vi "PLC_OP10_Read.vi"(8 "error in (no error)":errorcluster, 11 "S7 Connection in":T1) -> (0 "error out":errorcluster, 3 "S7 Connection out":T1)   [LabVIEW 2017]
uses:
  <vilib>/DATA AHEAD/SP7/typedefs/S7 Connection.ctl
  <vilib>/DATA AHEAD/SP7/typedefs/PLC Type.ctl
  <vilib>/DATA AHEAD/SP7/functions/read/read real array.vi
  <vilib>/DATA AHEAD/SP7/functions/read/read String.vi
  <vilib>/DATA AHEAD/SP7/functions/read/read Dint array.vi
  <vilib>/DATA AHEAD/SP7/SP7.lvlib
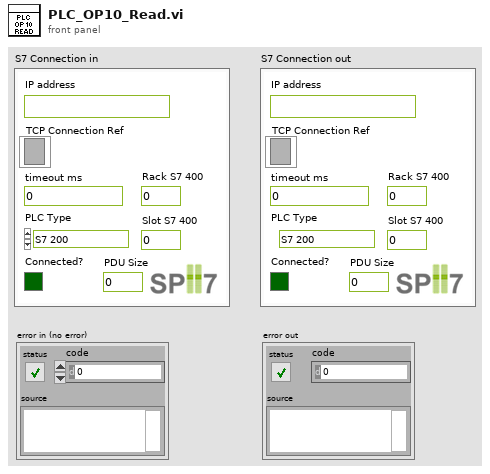
[diagram p1: front panel]
types:
  T1 = typedef "SP7.lvlib/S7 Connection.ctl" = cluster{"TCP Connection Ref":refnum<k5>, "IP address":string, "timeout ms":i32, "Connected?":bool, "PLC Type":T2, "Rack S7 400":u8, "Slot S7 400":u8, "PDU Size":u16, "connection semaphore":T3}
  T2 = typedef "SP7.lvlib/PLC Type.ctl" = enum16{"S7 200", "S7 300/400", "S7 1200", "S7 1500", "LOGO!8"}
  T3 = typedef "Semaphore RefNum" = refnum<k1>
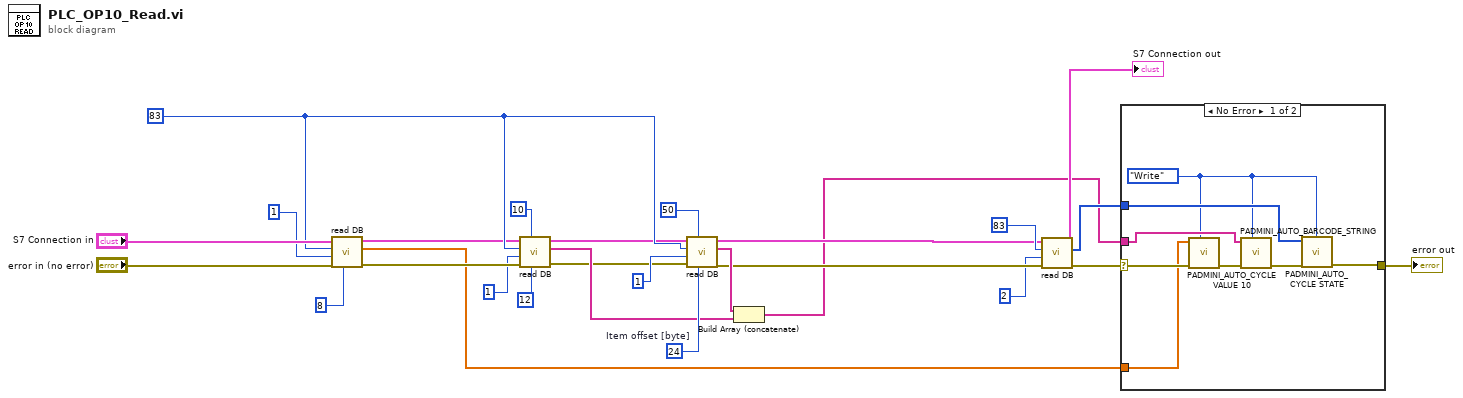
[diagram p0: block diagram]
diagram:
  w25 = u32 24  # Item offset [byte]
  w23 = u16 83 ("Data Block #")
  n1 = call-poly <vilib>:"read DB.vi"("Item offset [byte]"=u32 8, "error in (no error)"="error in (no error)", "items #"=u16 1 ("Items # [byte]"), "Data Block #"=w23, "S7 Connection in"="S7 Connection in") -> ("error out"=w15:errorcluster, "REAL result array"=w1:sgl[], "S7 Connection out"=w11:T1)  [unwired: 4 in]
  n2 = call-poly <vilib>:"read DB.vi"("Item offset [byte]"=u32 12, "String length reserved in DB (default=254)"=u16 10, "error in (no error)"=w15, "items #"=u16 1 ("Items # [byte]"), "Data Block #"=w23, "S7 Connection in"=w11) -> ("error out"=w17:errorcluster, "STRING result Array"=w20:string[], "S7 Connection out"=w16:T1)  [unwired: 2 in, 1 out]
  n3 = call-poly <vilib>:"read DB.vi"("Item offset [byte]"=w25, "String length reserved in DB (default=254)"=u16 50, "error in (no error)"=w17, "items #"=u16 1 ("Items # [byte]"), "Data Block #"=w23, "S7 Connection in"=w16) -> ("error out"=w18:errorcluster, "STRING result Array"=w21:string[], "S7 Connection out"=w5:T1)  [unwired: 2 in, 1 out]
  n4 = Build Array (concatenate)(w21, w20) -> (w2:string[])
  n5 = call-poly <vilib>:"read DB.vi"("error in (no error)"=w18, "items #"=u16 2 ("Items # [byte]"), "Data Block #"=u16 83, "S7 Connection in"=w5) -> ("error out"=w9:errorcluster, "DINT result array"=w7:i32[], "S7 Connection out"=→"S7 Connection out":T1)  [unwired: 5 in]
  n6 = case shown="No Error" w9 {
    selector: w9 -> [w31 w36]
    tunnel: w7 -> [w35 _]
    tunnel: [w34 w36] -> w3
    tunnel: w2 -> [w32 _]
    tunnel: w1 -> [w28 _]
    frame No Error {
      w29 = enum16{"Read", "Write"}."Write" ("Enum")
      n7 = call "PADMINI_AUTO_CYCLE VALUE 10.vi"("Enum"=w29, "error in (no error)"=w31, "Input"=w28) -> ("error out"=w30:errorcluster)  [unwired: 7 in, 1 out]
      n8 = call "PADMINI_AUTO_BARCODE_STRING.vi"("Enum"=w29, "error in (no error)"=w30, "Input"=w32) -> ("error out"=w33:errorcluster)  [unwired: 7 in, 1 out]
      n9 = call "PADMINI_AUTO_CYCLE STATE.vi"("Enum"=w29, "error in (no error)"=w33, "Input"=w35) -> ("error out"=w34:errorcluster)  [unwired: 7 in, 1 out]
    }
    frame Error {
    }
  }
  "error out" <- w3
